vi "Create Tags.vi"(6 "Overwrite Duplicates? (F)":bool, 8 "error in (no error)":errorcluster, 10 "Clear Table? (F)":bool, 11 "CVT Tags to Create":T1) -> (0 "error out":errorcluster)   [LabVIEW 2010, in "Current Value Table.lvlib"]
doc: "This VI loads CVT3 tags into the CVT."
uses:
  Current Value Table.lvlib
  Type Defs/File Format.ctl
  Type Defs/Single Tag.ctl
  Type Defs/Data Types.ctl
  Type Defs/Tag Grouping set.ctl
  FGVs/Tag Memory Methods.ctl
  Clear All Memory Blocks.vi
  Memory Block.vi
  DataTypes/Array of String_Memory Block.vi
  DataTypes/Array of Boolean_Memory Block.vi
  DataTypes/Array of Single_Memory Block.vi
  DataTypes/Array of Double_Memory Block.vi
  DataTypes/Array of I8_Memory Block.vi
  DataTypes/Array of I16_Memory Block.vi
  DataTypes/Array of I32_Memory Block.vi
  DataTypes/Array of I64_Memory Block.vi
  DataTypes/Array of U64_Memory Block.vi
  DataTypes/Array of U32_Memory Block.vi
  DataTypes/Array of U16_Memory Block.vi
  DataTypes/Array of U8_Memory Block.vi
  DataTypes/Boolean_Memory Block.vi
  DataTypes/String_Memory Block.vi
  DataTypes/U8_Memory Block.vi
  DataTypes/U16_Memory Block.vi
  DataTypes/U32_Memory Block.vi
  DataTypes/U64_Memory Block.vi
  DataTypes/I8_Memory Block.vi
  DataTypes/I16_Memory Block.vi
  DataTypes/I32_Memory Block.vi
  DataTypes/I64_Memory Block.vi
  DataTypes/Single_Memory Block.vi
  DataTypes/Double_Memory Block.vi
  FGVs/CVT Globals.vi
  FGVs/Group Memory.vi
  Form Single Group.vi
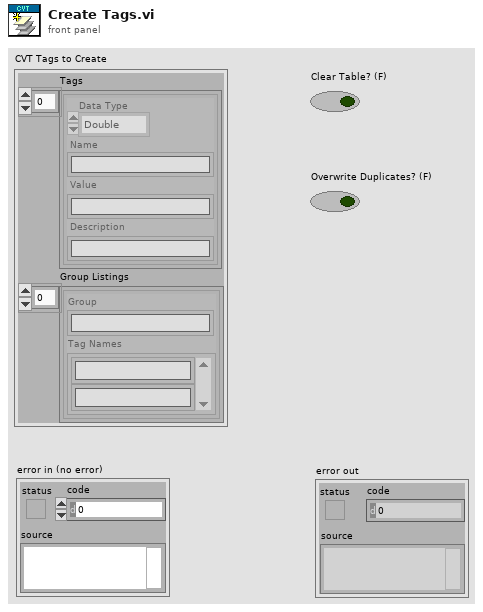
[diagram p1: front panel]
types:
  T1 = typedef "Current Value Table.lvlib/File Format.ctl" = cluster{"Tags":T2[], "Group Listings":T4[]}
  T2 = typedef "Current Value Table.lvlib/Single Tag.ctl" = cluster{"Data Type":T3, "Name":string, "Value":string, "Description":string}
  T3 = typedef "Current Value Table.lvlib/Data Types.ctl" = enum16{"Double", "Single", "I64", "I32", "I16", "I8", "U64", "U32", "U16", "U8", "String", "Boolean", "Array of U8", "Array of U16", "Array of U32", "Array of U64", "Array of I64", "Array of I32", "Array of I16", "Array of I8", "Array of Double", "Array of Single", "Array of Boolean", "Array of String"}
  T4 = typedef "Current Value Table.lvlib/Tag Grouping set.ctl" = cluster{"Group":string, "Tag Names":string[]}
  T5 = typedef "Current Value Table.lvlib/Tag Memory Methods.ctl" = enum16{"Clear", "Read Tag Index", "Read Tag Indices", "Generate Group", "Add Tag", "Overwrite Tag", "Read Description", "Get Stored Tags"}
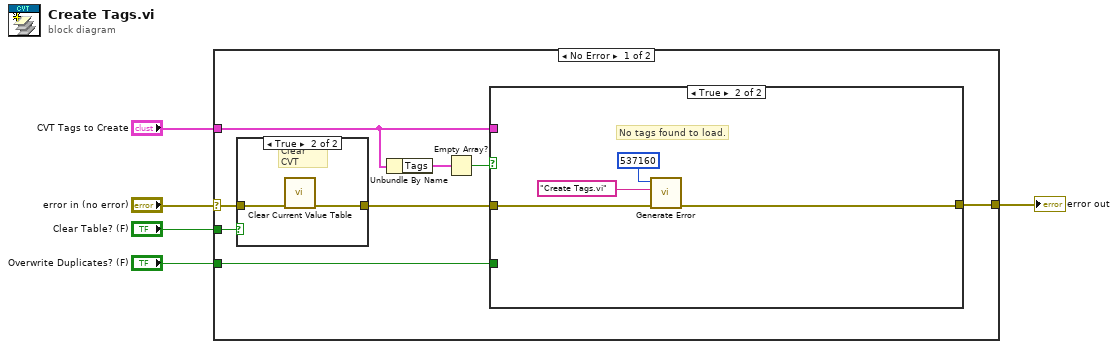
[diagram p0: block diagram]
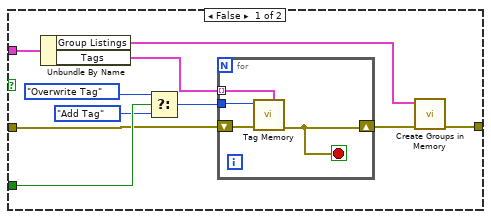
[diagram p2: hidden frame]
diagram:
  n1 = case shown="No Error" "error in (no error)" {
    selector: "error in (no error)" -> [w8 w35]
    tunnel: [w13 w35] -> w5
    tunnel: "Clear Table? (F)" -> [w12 _]
    tunnel: "Overwrite Duplicates? (F)" -> [w11 _]
    tunnel: "CVT Tags to Create" -> [w9 _]
    frame No Error {
      n2 = case shown="True" w12 {
        tunnel: [w32 w33] -> w7
        tunnel: w8 -> [w32 w34]
        frame False {
          # "Add tags"
        }
        frame True {
          # "Clear CVT"
          n3 = call "Clear Current Value Table.vi"("error in (no error)"=w34) -> ("error out"=w33:errorcluster)  [unwired: 10 in]
        }
      }
      n4 = Unbundle By Name(w9) -> ("Tags"=w10:T2[])
      n5 = Empty Array?(array=w10) -> (empty?=w6:bool)
      n6 = case shown="True" w6 {
        tunnel: w9 -> [w23 _]
        tunnel: [w21 w28] -> w13
        tunnel: w11 -> [w19 _]
        tunnel: w7 -> [w14 w29]
        frame False {
          n7 = Unbundle By Name(w23) -> ("Group Listings"=w22:T4[], "Tags"=w20:T2[])
          n8 = Select(t=Tag_Memory_Methods."Overwrite Tag" ("Method"), s=w19, f=Tag_Memory_Methods."Add Tag" ("Method")) -> (s? t:f=w16:T5)
          n9 = for {
            tunnel: w20 -> [w26] mode=indexing
            tunnel: w16 -> [w27]
            shift-right: [w25] -> w15
            shift-left: w14 -> [w24]
            stop <- w25 stop-if-true
            n10 = call "Tag Memory.vi"("Tag In"=w26, "error in (no error)"=w24, "Method"=w27) -> ("error out"=w25:errorcluster)  [unwired: 3 in, 5 out]
          }
          n11 = call "Create Groups in Memory.vi"("error in (no error)"=w15, "Group Listings"=w22) -> ("error out"=w21:errorcluster)  [unwired: 9 in]
        }
        frame True {
          # "No tags found to load."
          n12 = call "Generate Error.vi"("error in"=w29, "caller name"="Create Tags.vi" ("caller VI name"), "code"=537160) -> ("error out"=w28:errorcluster)  [unwired: 8 in]
        }
      }
    }
    frame Error {
    }
  }
  "error out" <- w5
